vi "Record Stage Data_YCC.vi"(3 "Save Data?":bool, 4 "Axis":u32=1, 5 "Record time (s)":u32=100) -> (0 "All Data (um)":dbl[](array[numeric]), 1 "mean now precise position (nm)":dbl format="%0.5f")   [LabVIEW 2014]
uses:
  (Global) Current handle and LaserPower_YCC.vi
  <vilib>/Utility/file.llb/Write To Spreadsheet File (DBL).vi
  MCL-dll-Labview 32-bit/Madlib.dll
  <vilib>/Analysis/NI_AALBase.lvlib
panel:
  in  "Tab Control":enum32{"Page 1", "Trace"}(tab)
  out "Histogram Graph":T1(graph)
  out "XY Graph":cluster{dbl[], dbl[]}(graph)
  out "Sampling Rate (Hz)":dbl
  in  "intervals":i32=10
  out "standard deviation (nm)":dbl format="%0.2f"
  in  "ADC Rate for 20bit (ms)":T2(ring)=enum."3750 Hz"
  # "3 -> 267us, 4 -> 500us , 5 -> 1ms , 6 -> 2ms, 7 -> 10ms , 8 -> 17ms , 9 -> 20ms"
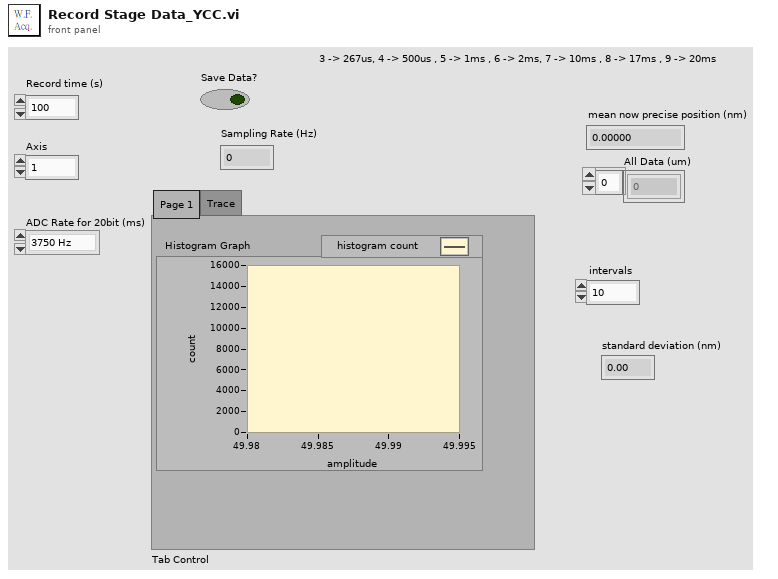
[diagram p1: front panel]
types:
  T1 = cluster{"X Values":dbl[], "Histogram: h(x)":i32[]}
  T2 = enum16{"50 Hz", "60 Hz", "100 Hz", "500 Hz", "1000 Hz", "2000 Hz", "3750 Hz"}
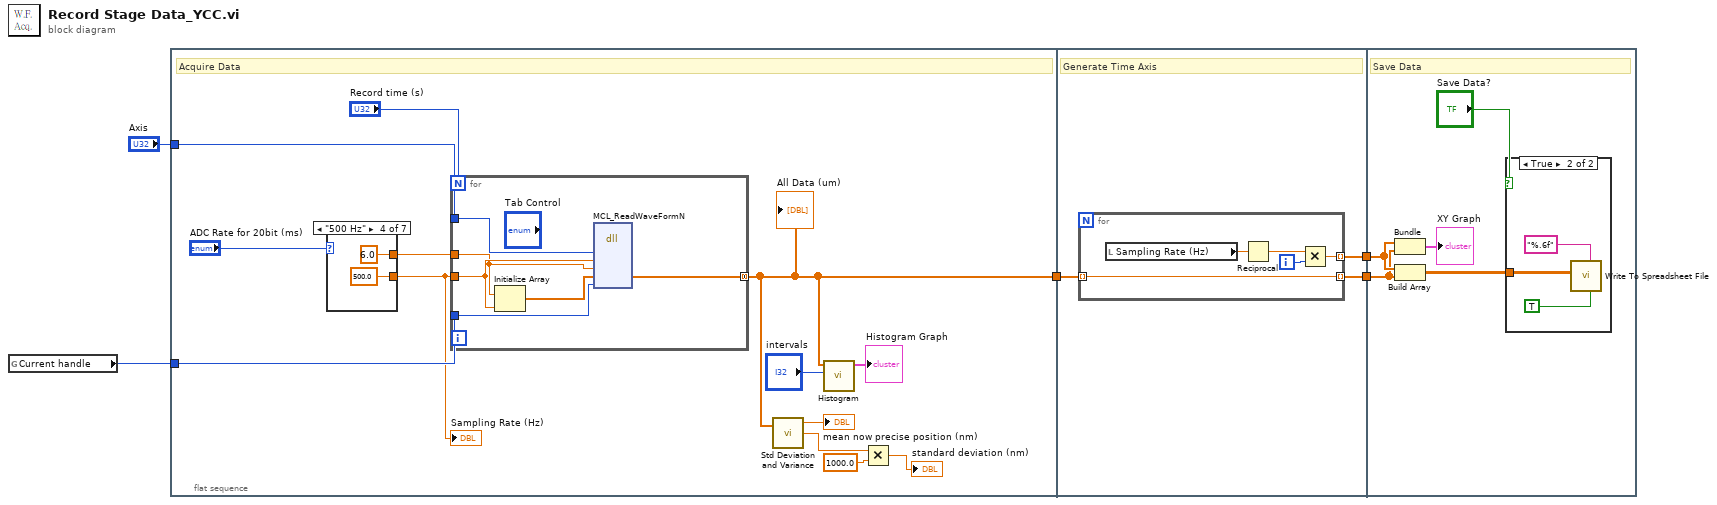
[diagram p0: block diagram]
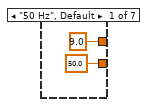
[diagram p2: hidden frame]
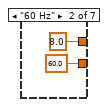
[diagram p3: hidden frame]
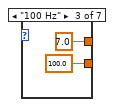
[diagram p4: hidden frame]
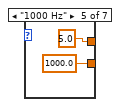
[diagram p5: hidden frame]
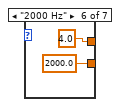
[diagram p6: hidden frame]
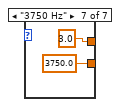
[diagram p7: hidden frame]
diagram:
  n1 = global read "(Global) Current handle and LaserPower_YCC.vi" "Current handle"() -> (w4:i32)
  n2 = flat-sequence {
    tunnel: "Axis" -> [w10]
    tunnel: w4 -> [w9]
    tunnel: [w6] -> w3
    tunnel: w3 -> [w41]
    tunnel: [w40] -> w2
    tunnel: [w39] -> w1
    tunnel: w2 -> [w48]
    tunnel: w1 -> [w49]
    frame #0 {
      # "Acquire Data"
      n3 = case shown="\"500 Hz\"" "ADC Rate for 20bit (ms)" {
        tunnel: [9.0 8.0 7.0 6.0 5.0 4.0 3.0] -> w17
        tunnel: [50.0 60.0 100.0 500.0 1000.0 2000.0 3750.0] -> w8
        frame "50 Hz", Default {
        }
        frame "60 Hz" {
        }
        frame "100 Hz" {
        }
        frame "500 Hz" {
        }
        frame "1000 Hz" {
        }
        frame "2000 Hz" {
        }
        frame "3750 Hz" {
        }
      }
      "Sampling Rate (Hz)" <- w8
      n4 = for {
        N: "Record time (s)" -> [_]
        tunnel: [w37] -> w6 mode=concatenating
        tunnel: w8 -> [w36]
        tunnel: w17 -> [w35]
        tunnel: w10 -> [w33]
        tunnel: w9 -> [w34]
        n5 = Initialize Array "Initialize Array"(w35, w36) -> (w38:dbl[])
        n6 = dll-call lib="C:/Users/OT-hwlab/Desktop/YCC's OT/Main-Stage-Based/SubVI-Stage-Based/MCL-dll-Labview 32-bit/MADLib.dll" fn="MCL_ReadWaveFormN"("axis"=w33, "DataPoints"=w36, "milliseconds"=w35, "waveform"=w38, "handle"=w34) -> ("waveform"=w37:dbl[])  [unwired: 8 in, 2 out]
      }
      "All Data (um)" <- w6
      n7 = call <vilib>:"Std Deviation and Variance.vi"("X"=w6) -> ("mean"=→"mean now precise position (nm)":dbl, "standard deviation"=w15:dbl)  [unwired: 1 in, 1 out]
      n8 = call <vilib>:"Histogram.vi"("intervals"="intervals", "X"=w6) -> ("Histogram Graph"=→"Histogram Graph":T1)  [unwired: 6 in, 3 out]
      n9 = Multiply(x=w15, y=1000.0) -> (x*y=→"standard deviation (nm)":dbl)
    }
    frame #1 {
      # "Generate Time Axis"
      n10 = for {
        tunnel: w41 -> [w46] mode=indexing
        tunnel: [w46] -> w40 mode=indexing
        tunnel: [w42] -> w39 mode=indexing
        i -> [w43]
        n11 = local read "Sampling Rate (Hz)"() -> (w45:dbl)
        n12 = Reciprocal(x=w45) -> (1/x=w44:dbl)
        n13 = Multiply(x=w44, y=w43) -> (x*y=w42:dbl)
      }
    }
    frame #2 {
      # "Save Data"
      n14 = Bundle(w49, w48) -> (→"XY Graph":cluster{dbl[], dbl[]})  [unwired: 1 in]
      n15 = Build Array(w49, w48) -> (w47:dbl[][])
      n16 = case shown="True" "Save Data?" {
        tunnel: w47 -> [_ w52]
        frame False {
        }
        frame True {
          n17 = call-poly <vilib>:"Write To Spreadsheet File.vi"("transpose? (no:F)"=TRUE, "format (%.3f)"="%.6f", "2D data"=w52) -> ()  [unwired: 5 in, 1 out]
        }
      }
    }
  }
